vi "SpeedSimulator.vi"(7 "Period":u32, 8 "error in":errorcluster, 10 "Brake":dbl, 11 "Gas":dbl) -> (0 "error out":errorcluster, 2 "Distance":dbl, 3 "Speed":dbl)   [LabVIEW 2012]
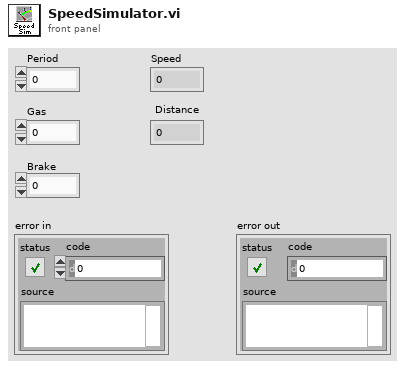
[diagram p1: front panel]
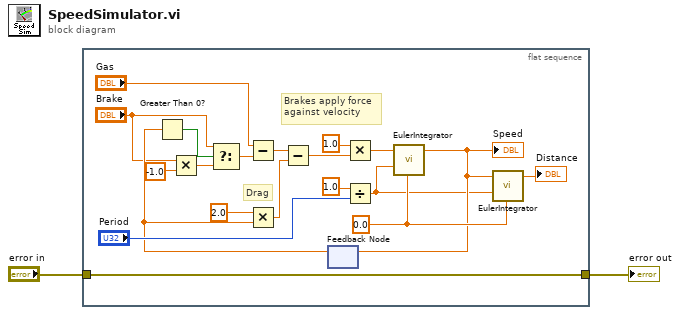
[diagram p0: block diagram]
diagram:
  n1 = flat-sequence {
    tunnel: "error in" -> [w3]
    tunnel: [w3] -> w1
    frame #0 {
      w21 = 0.0
      # "Brakes apply force\nagainst velocity"
      # "Drag"
      n2 = Multiply(x="Brake", y=-1.0) -> (x*y=w6:dbl)
      n3 = feedback #1() -> (w9:dbl)  [unwired: 1 in]
      n4 = Greater Than 0?(x=w9) -> (x > 0?=w8:bool)
      n5 = Select(t="Brake", s=w8, f=w6) -> (s? t:f=w7:dbl)
      n6 = Subtract(x="Gas", y=w7) -> (x-y=w16:dbl)
      n7 = Multiply(x=2.0, y=w9) -> (x*y=w15:dbl)
      n8 = Subtract(x=w16, y=w15) -> (x-y=w18:dbl)
      n9 = Multiply(x=1.0, y=w18) -> (x*y=w14:dbl)
      n10 = Divide(x=1.0, y="Period") -> (x/y=w11:dbl)
      n11 = call "EulerIntegrator.vi"("xDot"=w14, "dt"=w11, "xInitial"=w21) -> ("x"=w12:dbl)  [unwired: 24 in]
      "Speed" <- w12
      n12 = feedback-in #1(w12) -> ()
      n13 = call "EulerIntegrator.vi"("xDot"=w12, "dt"=w11, "xInitial"=w21) -> ("x"=→"Distance":dbl)  [unwired: 24 in]
    }
  }
  "error out" <- w1
